vi "butterscotch_test.vi"() -> ()   [LabVIEW 2012]
uses:
  <vilib>/Analysis/3filter.llb/Filter Passband Type.ctl
  <vilib>/Analysis/3filter.llb/Butterworth Filter (DBL).vi
  <vilib>/Analysis/NI_AALBase.lvlib
panel:
  out "Filtered X":dbl[][](array[numeric])
  out "readout (voltage or current)":waveform(dbl)[](graph)
  in  "file path":path
  in  "sampling freq: fs":dbl=1.0 format="%0.2f"
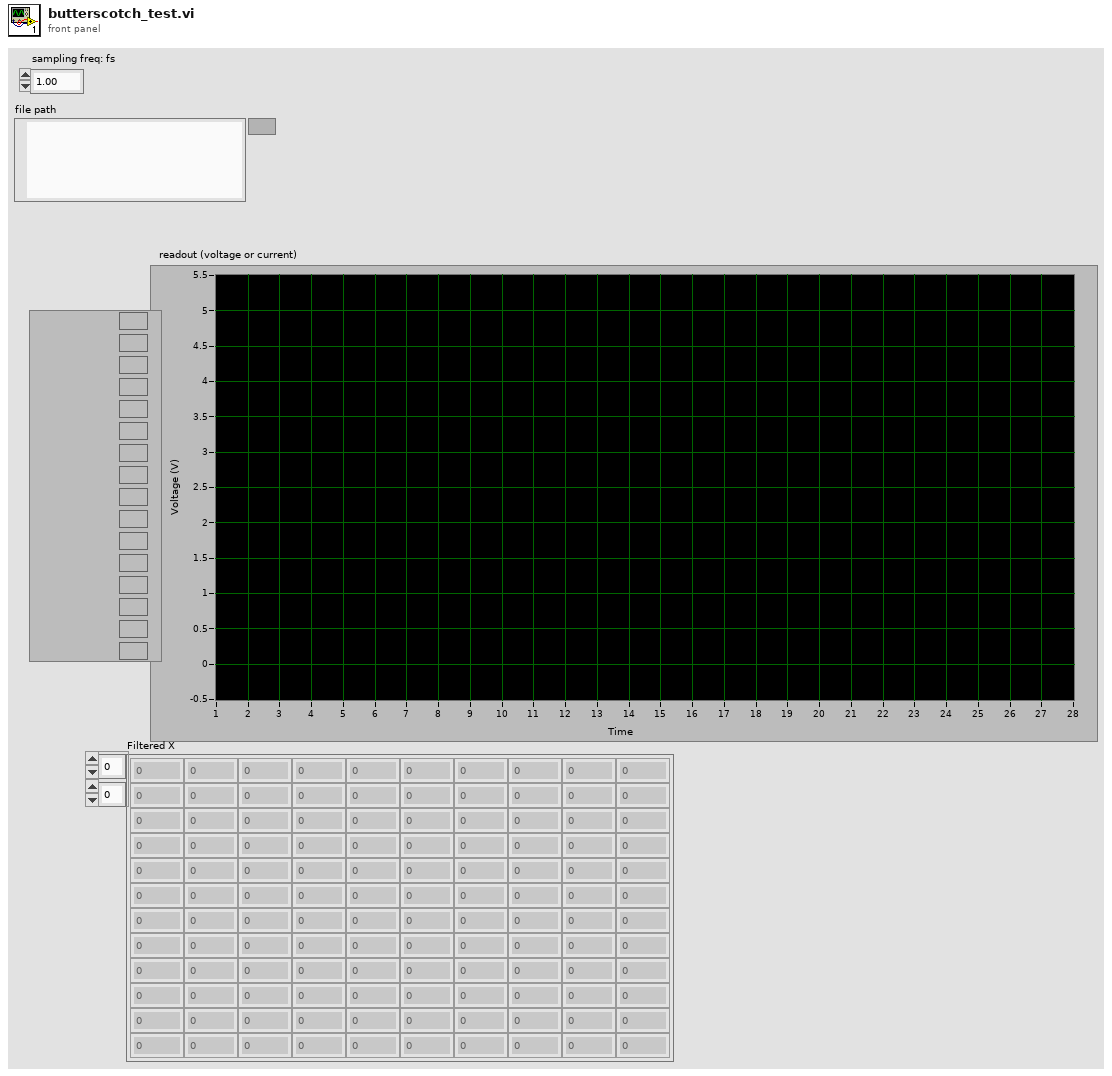
[diagram p1: front panel]
types:
  T1 = typedef "NI_AALBase.lvlib/Filter Passband Type.ctl" = enum32{"Lowpass", "Highpass", "Bandpass", "Bandstop"}
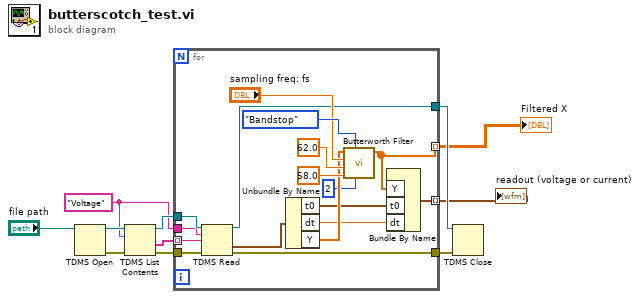
[diagram p0: block diagram]
diagram:
  w3 = "Voltage" ("group name")
  n1 = TDMS Open(11:"file path") -> (0:w9:errorcluster, 3:w10:refnum<k34>)  [unwired: 5 in]
  n2 = TDMS List Contents(4:w9, 6:w3, 7:w10) -> (0:w8:errorcluster, 1:w5:string[], 3:w7:refnum<k34>)  [unwired: 1 out]
  n3 = for {
    tunnel: w8 -> [w24]
    tunnel: w7 -> [w23]
    tunnel: [w22] -> w6
    tunnel: w5 -> [w21] mode=indexing
    tunnel: [w20] -> w4
    tunnel: w3 -> [w19]
    tunnel: [w14] -> w2 mode=indexing
    tunnel: [w13] -> w1 mode=indexing
    n4 = TDMS Read(0:w23, 5:w19, 7:w21, 11:w24) -> (4:w22:refnum<k34>, 10:w18:waveform(dbl), 15:w20:errorcluster)  [unwired: 4 in, 3 out]
    n5 = Unbundle By Name(w18) -> ("t0"=w16:timestamp, "dt"=w15:dbl, "Y"=w17:dbl[])
    n6 = call-poly <vilib>:"Butterworth Filter.vi"("order"=2, "filter type"=Filter_Passband_Type."Bandstop", "low cutoff freq: fl"=58.0, "high cutoff freq: fh"=62.0, "sampling freq: fs"="sampling freq: fs", "X"=w17) -> ("Filtered X"=w13:dbl[])  [unwired: 2 in, 1 out]
    n7 = Bundle By Name("Y"=w13, "t0"=w16, "dt"=w15) -> (w14:waveform(dbl))  [unwired: 1 in]
  }
  "readout (voltage or current)" <- w2
  "Filtered X" <- w1
  n8 = TDMS Close(8:w4, 11:w6) -> ()  [unwired: 2 out]
